vi "TestSquare.vi"() -> ()   [LabVIEW 2013]
uses:
  <vilib>/measure/NI_MABase.lvlib
panel:
  in  "Components":i32=3
  in  "Amp":dbl=10.0 format="%#_13g"
  in  "sampling info":cluster{"Fs":dbl, "#s":dbl}={"Fs"=100.0, "#s"=1600.0}
  in  "frequency":dbl=0.0625 format="%#_13g"
  out "Decomposed":dbl[](array[numeric])
  out "Eye Vel":dbl[][](graph)
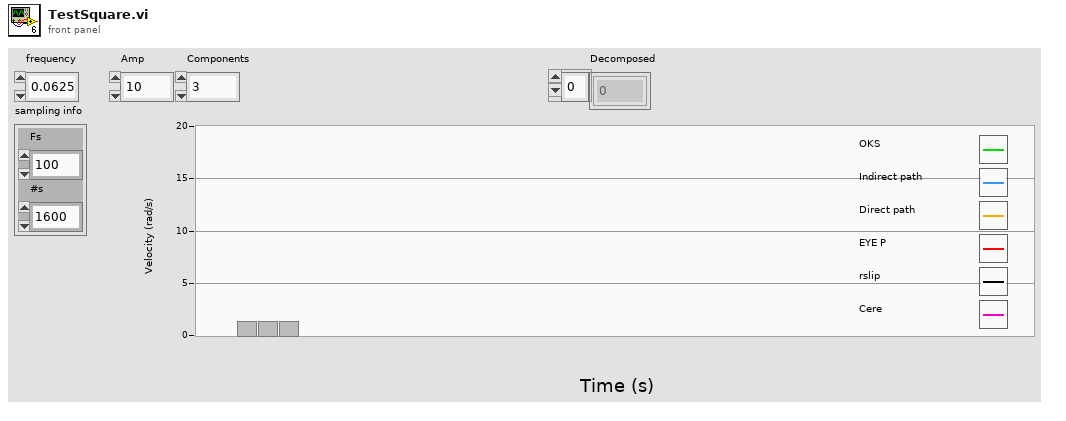
[diagram p1: front panel]
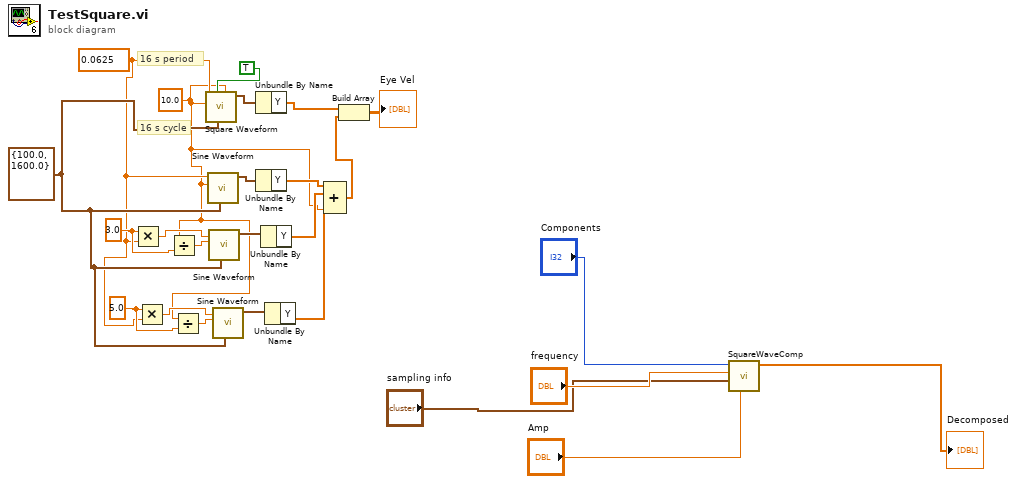
[diagram p0: block diagram]
diagram:
  w16 = 5.0 ("x")
  w17 = 3.0 ("x")
  w12 = cluster{"Fs":dbl, "#s":dbl} {"Fs"=100.0, "#s"=1600.0} ("sampling info")
  w8 = 0.0625 ("frequency")
  w7 = 10.0 ("offset")
  # "16 s period"
  # "16 s cycle"
  n1 = Multiply(x=w17, y=w8) -> (x*y=w21:dbl)
  n2 = Multiply(x=w16, y=w8) -> (x*y=w13:dbl)
  n3 = Divide(x=w7, y=w17) -> (x/y=w18:dbl)
  n4 = Divide(x=w7, y=w16) -> (x/y=w15:dbl)
  n5 = call <vilib>:"Square Waveform.vi"("offset"=w7, "sampling info"=w12, "reset signal"=TRUE, "amplitude"=w7, "frequency"=w8) -> ("signal out"=w19:waveform(dbl))  [unwired: 5 in, 1 out]
  n6 = call <vilib>:"Sine Waveform.vi"("sampling info"=w12, "amplitude"=w7, "frequency"=w8) -> ("signal out"=w22:waveform(dbl))  [unwired: 7 in, 1 out]
  n7 = call <vilib>:"Sine Waveform.vi"("sampling info"=w12, "amplitude"=w18, "frequency"=w21) -> ("signal out"=w20:waveform(dbl))  [unwired: 7 in, 1 out]
  n8 = call <vilib>:"Sine Waveform.vi"("sampling info"=w12, "amplitude"=w15, "frequency"=w13) -> ("signal out"=w14:waveform(dbl))  [unwired: 7 in, 1 out]
  n9 = Unbundle By Name(w19) -> ("Y"=w24:dbl[])
  n10 = Unbundle By Name(w22) -> ("Y"=w11:dbl[])
  n11 = Unbundle By Name(w20) -> ("Y"=w10:dbl[])
  n12 = Unbundle By Name(w14) -> ("Y"=w3:dbl[])
  n13 = Compound Arithmetic op=ADD(w11, w10, w3, w7) -> (w9:dbl[])
  n14 = Build Array(w24, w9) -> (→"Eye Vel":dbl[][])
  n15 = call "SquareWaveComp.vi"("Amp"="Amp", "sampling info"="sampling info", "frequency"="frequency", "Components"="Components") -> ("Decomposed"=→"Decomposed":dbl[])  [unwired: 7 in]
